vi "inspectionForm.vi"() -> ()   [LabVIEW 2018]
uses:
  MotorController/#include/Global textParse.vi
panel:
  in  "Device Type":bool caption="Boolean"
  out "Initialize":string
  in  "E-Stop":bool
  in  "SpecSheet Scan":string
  in  "VISA Oscilloscope 2":refnum<visa-resource-name>
  in  "VISA Oscilloscope 1":refnum<visa-resource-name>
  in  "Serial Port":refnum<visa-resource-name>
  in  "Number of Oscilloscopes":bool caption="Boolean"
  in  "PO Line#":string
  in  "PO#":string
  in  "Number":string
  in  "Vendor":string
  in  "Station":string
  in  "Inspector":string
  in  "Inspection Point":string(combo)
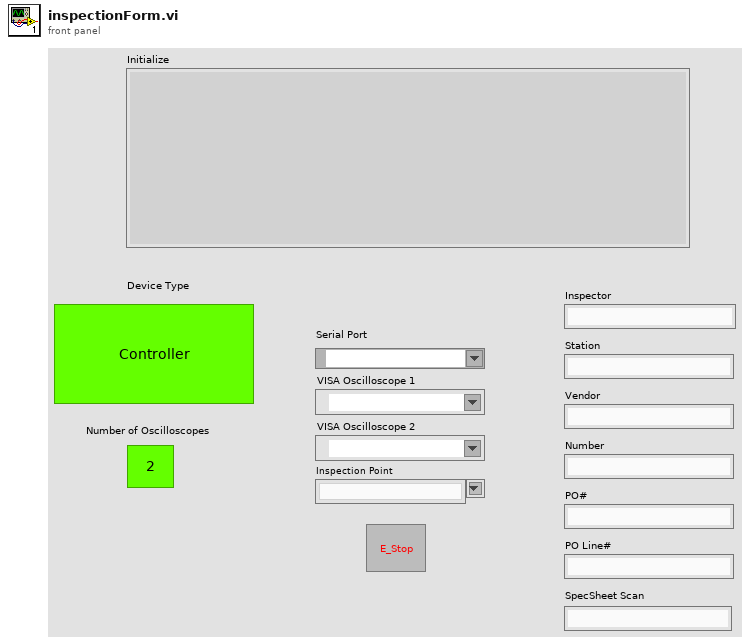
[diagram p1: front panel]
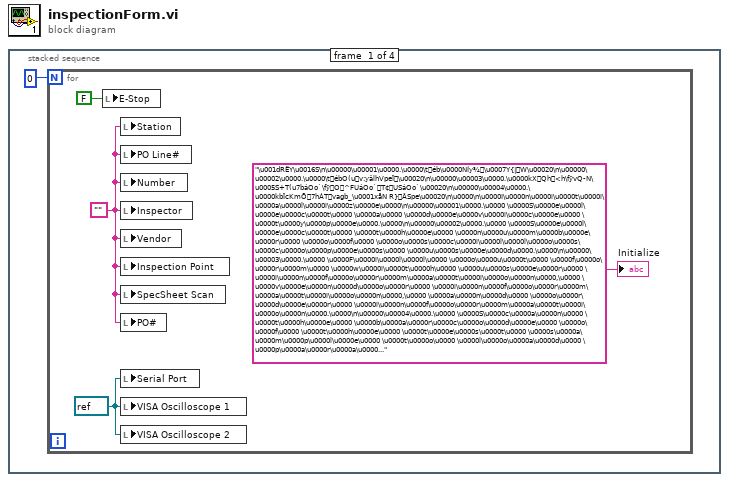
[diagram p0: block diagram]
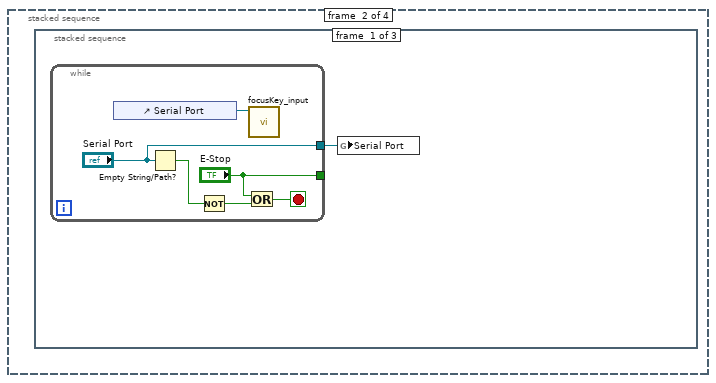
[diagram p2: hidden frame]
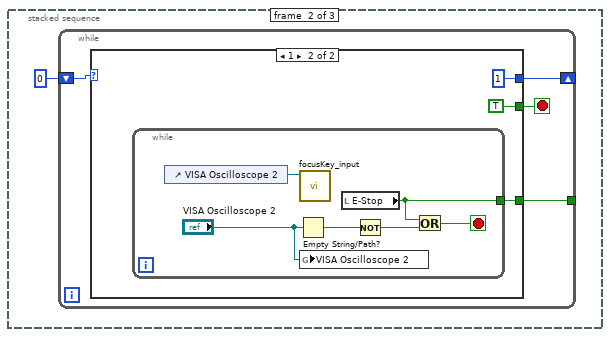
[diagram p3: hidden frame]
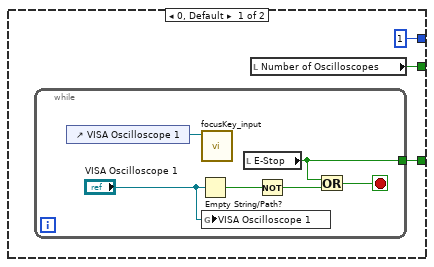
[diagram p4: hidden frame]
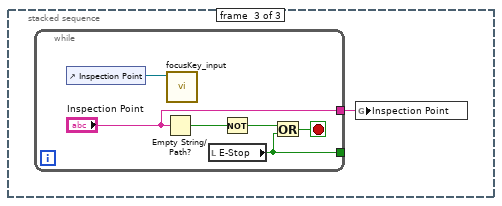
[diagram p5: hidden frame]
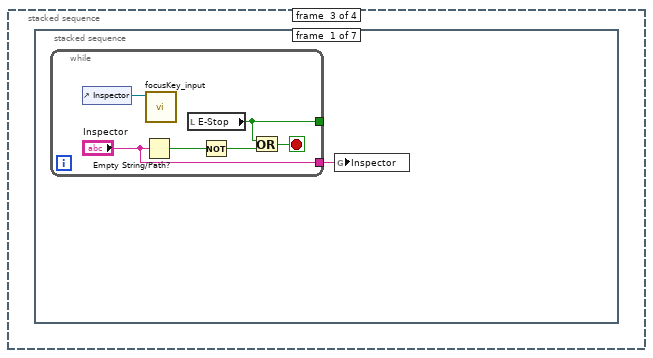
[diagram p6: hidden frame]
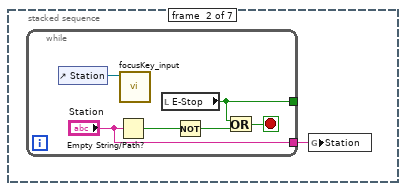
[diagram p7: hidden frame]
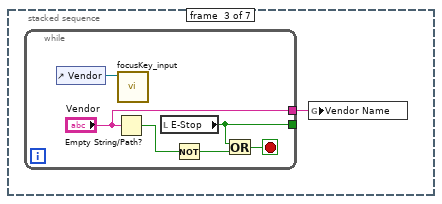
[diagram p8: hidden frame]
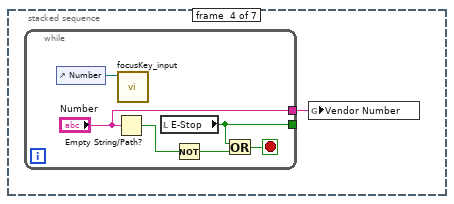
[diagram p9: hidden frame]
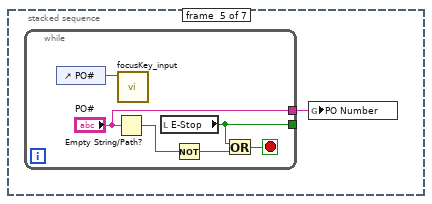
[diagram p10: hidden frame]
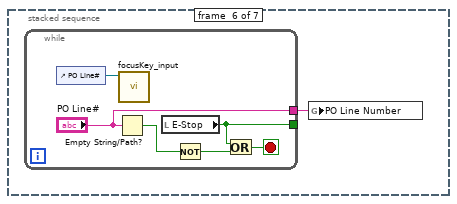
[diagram p11: hidden frame]
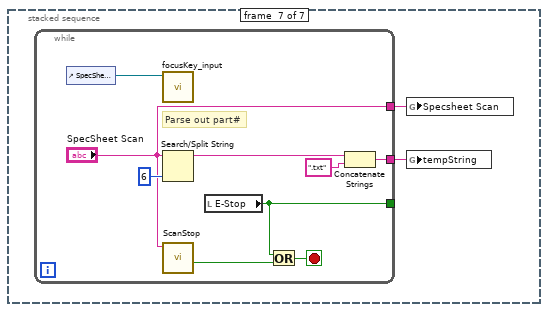
[diagram p12: hidden frame]
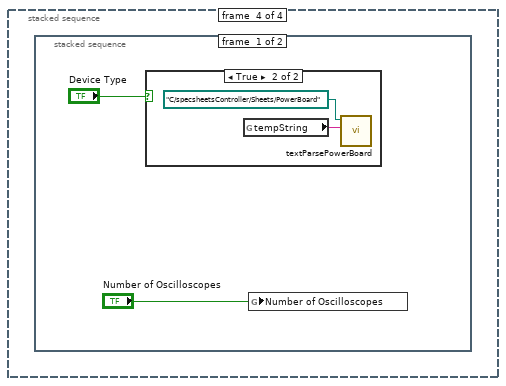
[diagram p13: hidden frame]
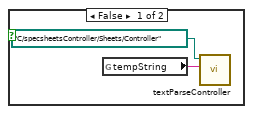
[diagram p14: hidden frame]
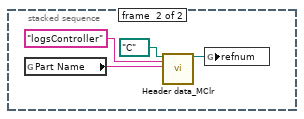
[diagram p15: hidden frame]
diagram:
  n1 = stacked-sequence {
    frame #0 {
      n2 = for {
        N: 0 -> [_]
        w3 = ""
        w4 = refnum<visa-resource-name> refnum ("VISA Oscilloscope 1")
        n3 = local write "E-Stop"(FALSE ("E-Stop")) -> ()
        n4 = local write "Station"(w3) -> ()
        n5 = local write "PO Line#"(w3) -> ()
        n6 = local write "Number"(w3) -> ()
        n7 = local write "Inspector"(w3) -> ()
        n8 = local write "Vendor"(w3) -> ()
        n9 = local write "Inspection Point"(w3) -> ()
        n10 = local write "SpecSheet Scan"(w3) -> ()
        n11 = local write "PO#"(w3) -> ()
        n12 = local write "Serial Port"(w4) -> ()
        n13 = local write "VISA Oscilloscope 1"(w4) -> ()
        n14 = local write "VISA Oscilloscope 2"(w4) -> ()
        "Initialize" <- "\u001dRËY\u0016S\n\u00000\u00001\u0000.\u0000\téb\u0000NÍy¾\u0007Y{|W\u00020\n\u00000\u00002\u0000.\u0000\tébO(uv:yâlhVpeÏ\u00020\n\u00000\u00003\u0000.\u0000kXQh<h\fÿvQ-N\u0005S+T(u7báOo`\fÿO^FUáOo`T¢USáOo`\u00020\n\u00000\u00004\u0000.\u0000kbÏcKmÕ7hÁTvagb_\u0001xåN R}ÂSpe\u00020\n\u0000\n\u0000I\u0000n\u0000i\u0000t\u0000i\u0000a\u0000l\u0000i\u0000z\u0000e\u0000\n\u00000\u00001\u0000.\u0000 \u0000S\u0000e\u0000l\u0000e\u0000c\u0000t\u0000 \u0000a\u0000 \u0000d\u0000e\u0000v\u0000i\u0000c\u0000e\u0000 \u0000t\u0000y\u0000p\u0000e\u0000.\u0000\n\u00000\u00002\u0000.\u0000 \u0000S\u0000e\u0000l\u0000e\u0000c\u0000t\u0000 \u0000t\u0000h\u0000e\u0000 \u0000n\u0000u\u0000m\u0000b\u0000e\u0000r\u0000 \u0000o\u0000f\u0000 \u0000o\u0000s\u0000c\u0000i\u0000l\u0000l\u0000o\u0000s\u0000c\u0000o\u0000p\u0000e\u0000s\u0000 \u0000u\u0000s\u0000e\u0000d\u0000.\u0000\n\u00000\u00003\u0000.\u0000 \u0000F\u0000i\u0000l\u0000l\u0000 \u0000o\u0000u\u0000t\u0000 \u0000f\u0000o\u0000r\u0000m\u0000 \u0000w\u0000i\u0000t\u0000h\u0000 \u0000u\u0000s\u0000e\u0000r\u0000 \u0000i\u0000n\u0000f\u0000o\u0000r\u0000m\u0000a\u0000t\u0000i\u0000o\u0000n\u0000,\u0000 \u0000v\u0000e\u0000n\u0000d\u0000o\u0000r\u0000 \u0000i\u0000n\u0000f\u0000o\u0000r\u0000m\u0000a\u0000t\u0000i\u0000o\u0000n\u0000,\u0000 \u0000a\u0000n\u0000d\u0000 \u0000o\u0000r\u0000d\u0000e\u0000r\u0000 \u0000i\u0000n\u0000f\u0000o\u0000r\u0000m\u0000a\u0000t\u0000i\u0000o\u0000n\u0000.\u0000\n\u00000\u00004\u0000.\u0000 \u0000S\u0000c\u0000a\u0000n\u0000 \u0000t\u0000h\u0000e\u0000 \u0000b\u0000a\u0000r\u0000c\u0000o\u0000d\u0000e\u0000 \u0000o\u0000f\u0000 \u0000t\u0000h\u0000e\u0000 \u0000t\u0000e\u0000s\u0000t\u0000 \u0000s\u0000a\u0000m\u0000p\u0000l\u0000e\u0000 \u0000t\u0000o\u0000 \u0000l\u0000o\u0000a\u0000d\u0000 \u0000p\u0000a\u0000r\u0000a\u0000..."
      }
    }
    frame #1 {
      n15 = stacked-sequence {
        frame #0 {
          n16 = while {
            tunnel: ["E-Stop"] -> _
            tunnel: ["Serial Port"] -> w6
            stop <- w9 stop-if-true
            n17 = control-ref of="Serial Port"() -> (w11:refnum<vi>)
            n18 = Empty String/Path?(string/path="Serial Port") -> (empty?=w12:bool)
            n19 = Not(x=w12) -> (.not. x?=w10:bool)
            n20 = Or(x="E-Stop", y=w10) -> (x .or. y?=w9:bool)
            n21 = call "focusKey_input.vi"("reference"=w11) -> ()  [unwired: 10 in, 1 out]
          }
          n22 = global write "Global textParse.vi" "Serial Port"(w6) -> ()
        }
        frame #1 {
          n23 = while {
            shift-right: [w14] -> _
            shift-left: 0 -> [w17]
            tunnel: [w16] -> _
            stop <- w15 stop-if-true
            n24 = case shown="1" w17 {
              tunnel: [w18 w29] -> w16
              tunnel: [w20 TRUE] -> w15
              tunnel: [1 1] -> w14
              frame 0, Default {
                n25 = while {
                  tunnel: [w22] -> w18
                  stop <- w24 stop-if-true
                  n26 = control-ref of="VISA Oscilloscope 1"() -> (w25:refnum<vi>)
                  n27 = Empty String/Path?(string/path="VISA Oscilloscope 1") -> (empty?=w26:bool)
                  n28 = call "focusKey_input.vi"("reference"=w25) -> ()  [unwired: 10 in, 1 out]
                  n29 = global write "Global textParse.vi" "VISA Oscilloscope 1"("VISA Oscilloscope 1") -> ()
                  n30 = local read "E-Stop"() -> (w22:bool)
                  n31 = Not(x=w26) -> (.not. x?=w23:bool)
                  n32 = Or(x=w22, y=w23) -> (x .or. y?=w24:bool)
                }
                n33 = local read "Number of Oscilloscopes"() -> (w20:bool)
              }
              frame 1 {
                n34 = while {
                  tunnel: [w31] -> w29
                  stop <- w33 stop-if-true
                  n35 = control-ref of="VISA Oscilloscope 2"() -> (w34:refnum<vi>)
                  n36 = Empty String/Path?(string/path="VISA Oscilloscope 2") -> (empty?=w35:bool)
                  n37 = call "focusKey_input.vi"("reference"=w34) -> ()  [unwired: 10 in, 1 out]
                  n38 = global write "Global textParse.vi" "VISA Oscilloscope 2"("VISA Oscilloscope 2") -> ()
                  n39 = local read "E-Stop"() -> (w31:bool)
                  n40 = Not(x=w35) -> (.not. x?=w32:bool)
                  n41 = Or(x=w31, y=w32) -> (x .or. y?=w33:bool)
                }
              }
            }
          }
        }
        frame #2 {
          n42 = while {
            tunnel: [w38] -> _
            tunnel: ["Inspection Point"] -> w36
            stop <- w42 stop-if-true
            n43 = control-ref of="Inspection Point"() -> (w39:refnum<vi>)
            n44 = Empty String/Path?(string/path="Inspection Point") -> (empty?=w41:bool)
            n45 = call "focusKey_input.vi"("reference"=w39) -> ()  [unwired: 10 in, 1 out]
            n46 = local read "E-Stop"() -> (w38:bool)
            n47 = Not(x=w41) -> (.not. x?=w40:bool)
            n48 = Or(x=w40, y=w38) -> (x .or. y?=w42:bool)
          }
          n49 = global write "Global textParse.vi" "Inspection Point"(w36) -> ()
        }
      }
    }
    frame #2 {
      n50 = stacked-sequence {
        frame #0 {
          n51 = while {
            tunnel: ["Inspector"] -> w43
            tunnel: [w44] -> _
            stop <- w46 stop-if-true
            n52 = control-ref of="Inspector"() -> (w47:refnum<vi>)
            n53 = Empty String/Path?(string/path="Inspector") -> (empty?=w49:bool)
            n54 = call "focusKey_input.vi"("reference"=w47) -> ()  [unwired: 10 in, 1 out]
            n55 = local read "E-Stop"() -> (w44:bool)
            n56 = Not(x=w49) -> (.not. x?=w45:bool)
            n57 = Or(x=w44, y=w45) -> (x .or. y?=w46:bool)
          }
          n58 = global write "Global textParse.vi" "Inspector"(w43) -> ()
        }
        frame #1 {
          n59 = while {
            tunnel: ["Station"] -> w50
            tunnel: [w51] -> _
            stop <- w53 stop-if-true
            n60 = control-ref of="Station"() -> (w54:refnum<vi>)
            n61 = Empty String/Path?(string/path="Station") -> (empty?=w56:bool)
            n62 = call "focusKey_input.vi"("reference"=w54) -> ()  [unwired: 10 in, 1 out]
            n63 = local read "E-Stop"() -> (w51:bool)
            n64 = Not(x=w56) -> (.not. x?=w52:bool)
            n65 = Or(x=w51, y=w52) -> (x .or. y?=w53:bool)
          }
          n66 = global write "Global textParse.vi" "Station"(w50) -> ()
        }
        frame #2 {
          n67 = while {
            tunnel: ["Vendor"] -> w57
            tunnel: [w58] -> _
            stop <- w60 stop-if-true
            n68 = control-ref of="Vendor"() -> (w61:refnum<vi>)
            n69 = Empty String/Path?(string/path="Vendor") -> (empty?=w63:bool)
            n70 = call "focusKey_input.vi"("reference"=w61) -> ()  [unwired: 10 in, 1 out]
            n71 = local read "E-Stop"() -> (w58:bool)
            n72 = Not(x=w63) -> (.not. x?=w59:bool)
            n73 = Or(x=w58, y=w59) -> (x .or. y?=w60:bool)
          }
          n74 = global write "Global textParse.vi" "Vendor Name"(w57) -> ()
        }
        frame #3 {
          n75 = while {
            tunnel: ["Number"] -> w64
            tunnel: [w65] -> _
            stop <- w67 stop-if-true
            n76 = control-ref of="Number"() -> (w68:refnum<vi>)
            n77 = Empty String/Path?(string/path="Number") -> (empty?=w70:bool)
            n78 = call "focusKey_input.vi"("reference"=w68) -> ()  [unwired: 10 in, 1 out]
            n79 = local read "E-Stop"() -> (w65:bool)
            n80 = Not(x=w70) -> (.not. x?=w66:bool)
            n81 = Or(x=w65, y=w66) -> (x .or. y?=w67:bool)
          }
          n82 = global write "Global textParse.vi" "Vendor Number"(w64) -> ()
        }
        frame #4 {
          n83 = while {
            tunnel: ["PO#"] -> w71
            tunnel: [w72] -> _
            stop <- w74 stop-if-true
            n84 = control-ref of="PO#"() -> (w75:refnum<vi>)
            n85 = Empty String/Path?(string/path="PO#") -> (empty?=w77:bool)
            n86 = call "focusKey_input.vi"("reference"=w75) -> ()  [unwired: 10 in, 1 out]
            n87 = local read "E-Stop"() -> (w72:bool)
            n88 = Not(x=w77) -> (.not. x?=w73:bool)
            n89 = Or(x=w72, y=w73) -> (x .or. y?=w74:bool)
          }
          n90 = global write "Global textParse.vi" "PO Number"(w71) -> ()
        }
        frame #5 {
          n91 = while {
            tunnel: ["PO Line#"] -> w78
            tunnel: [w79] -> _
            stop <- w83 stop-if-true
            n92 = control-ref of="PO Line#"() -> (w81:refnum<vi>)
            n93 = Empty String/Path?(string/path="PO Line#") -> (empty?=w82:bool)
            n94 = call "focusKey_input.vi"("reference"=w81) -> ()  [unwired: 10 in, 1 out]
            n95 = local read "E-Stop"() -> (w79:bool)
            n96 = Not(x=w82) -> (.not. x?=w84:bool)
            n97 = Or(x=w79, y=w84) -> (x .or. y?=w83:bool)
          }
          n98 = global write "Global textParse.vi" "PO Line Number"(w78) -> ()
        }
        frame #6 {
          n99 = while {
            tunnel: ["SpecSheet Scan"] -> w86
            tunnel: [w91] -> w85
            tunnel: [w87] -> _
            stop <- w88 stop-if-true
            # "Parse out part#"
            n100 = control-ref of="SpecSheet Scan"() -> (w95:refnum<vi>)
            n101 = call "focusKey_input.vi"("reference"=w95) -> ()  [unwired: 10 in, 1 out]
            n102 = Search/Split String(string="SpecSheet Scan", offset (0)=6) -> (substring before match=w92:string)  [unwired: 1 in, 2 out]
            n103 = call "ScanStop.vi"("bar code scan"="SpecSheet Scan") -> ("Output"=w90:bool)  [unwired: 8 in, 2 out]
            n104 = local read "E-Stop"() -> (w87:bool)
            n105 = Or(x=w87, y=w90) -> (x .or. y?=w88:bool)
            n106 = Concatenate Strings(w92, ".txt" ("string")) -> (w91:string)
          }
          n107 = global write "Global textParse.vi" "Specsheet Scan"(w86) -> ()
          n108 = global write "Global textParse.vi" "tempString"(w85) -> ()
        }
      }
    }
    frame #3 {
      n109 = stacked-sequence {
        frame #0 {
          n110 = case shown="True" "Device Type" {
            frame False {
              n111 = global read "Global textParse.vi" "tempString"() -> (w99:string)
              n112 = call "textParseController.vi"("file name"=w99, "base path"=path "C:/specsheetsController/Sheets/Controller") -> ()  [unwired: 7 in, 3 out]
            }
            frame True {
              n113 = global read "Global textParse.vi" "tempString"() -> (w101:string)
              n114 = call "textParsePowerBoard.vi"("file name"=w101, "base path"=path "C:/specsheetsController/Sheets/PowerBoard") -> ()  [unwired: 7 in, 3 out]
            }
          }
          n115 = global write "Global textParse.vi" "Number of Oscilloscopes"("Number of Oscilloscopes") -> ()
        }
        frame #1 {
          n116 = global read "Global textParse.vi" "Part Name"() -> (w105:string)
          n117 = call "Header data_MClr.vi"("base path"=path "C:/", "prompt (Create Folder)"="logsController", "file name"=w105) -> ("refnum out"=w102:refnum<file>)  [unwired: 15 in, 1 out]
          n118 = global write "Global textParse.vi" "refnum"(w102) -> ()
        }
      }
    }
  }
